vi "GetType.vi"(8 "error in (no error)":errorcluster, 11 "Configure Trigger Slope [TS] Msg":refnum<class "Configure Trigger Slope [TS] Msg.lvclass">) -> (0 "error out":errorcluster, 2 "Data Sample":variant, 3 "Configure Trigger Slope [TS] Msg":refnum<class "Configure Trigger Slope [TS] Msg.lvclass">)   [LabVIEW 2015, in "CS++DMM.lvlib" / "Configure Trigger Slope [TS] Msg.lvclass"]
uses:
  Configure Trigger Slope [TS] Msg.lvclass
  Configure Trigger Slope [TS] Msg.lvclass/Configure Trigger Slope [TS] Msg.ctl
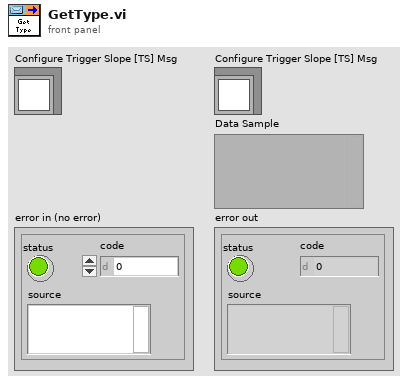
[diagram p1: front panel]
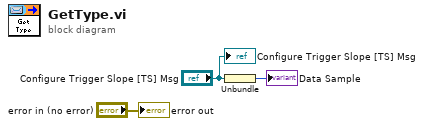
[diagram p0: block diagram]
diagram:
  n1 = Unbundle("Configure Trigger Slope [TS] Msg") -> (→"Data Sample":i32)
  "error out" <- "error in (no error)"
  "Configure Trigger Slope [TS] Msg" <- "Configure Trigger Slope [TS] Msg"
